vi "test.vi"() -> ()   [LabVIEW 2020]
uses:
  <vilib>/Instr/_visa.llb/VISA Configure Serial Port (Instr).vi
panel:
  out "nombre renvoyé":u32
  out "ERRIN":errorcluster caption="sortie d'erreur"
  in  "ERRIN":errorcluster caption="entrée d'erreur (pas d'erreur)"
  in  "VISA ST5520":refnum<visa-resource-name> caption="Nom de ressource VISA"
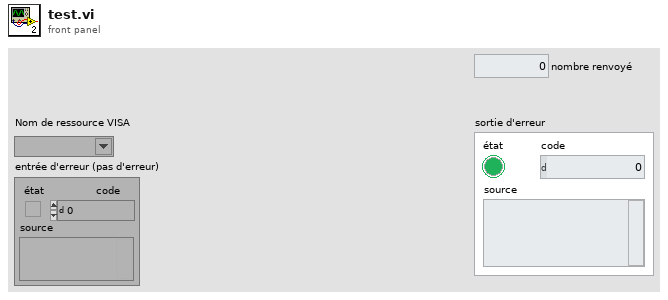
[diagram p1: front panel]
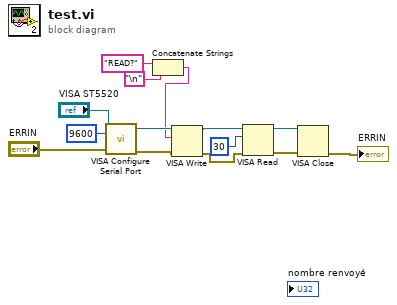
[diagram p0: block diagram]
diagram:
  n1 = call-poly "VISA Configure Serial Port"("VISA resource name"="VISA ST5520", "baud rate (9600)"=u32 9600, "error in (no error)"="ERRIN") -> ("VISA resource name out"=w8:refnum<visa-resource-name>, "error out"=w7:errorcluster)  [unwired: 11 in]
  n2 = Concatenate Strings("READ?" ("chaîne"), "\n") -> (w6:string)
  n3 = VISA Write(VISA resource name=w8, write buffer=w6, error in (no error)=w7) -> (VISA resource name out=w5:refnum<visa-resource-name>, error out=w3:errorcluster)  [unwired: 1 out]
  n4 = VISA Read(VISA resource name=w5, byte count=u32 30 ("nombre d'octets"), error in (no error)=w3) -> (VISA resource name out=w1:refnum<visa-resource-name>, error out=w2:errorcluster)  [unwired: 2 out]
  n5 = VISA Close(VISA resource name=w1, error in (no error)=w2) -> (error out=→"ERRIN":errorcluster)
